vi "CH_LM Config Speedup.vi"(0 "Meter Index":i32, 2 "Speedup Mode (0)":T1, 3 "Status (On)":bool=TRUE, 5 "error in (no error)":errorcluster, 7 "Timeout / ms (3000)":i32=3000, 8 "Action (query)":bool, 9 "Lock Timeout / ms (1000)":i32=1000) -> (11 "Lock timed out":bool, 14 "Meter Index":i32, 17 "Status":bool, 19 "error out":errorcluster)   [LabVIEW 2012, in "CH_LM.lvlib"]
doc: "This command will set/query speedup modes."
uses:
  CH_LM.lvlib
  CH_LM Speedup Type.ctl
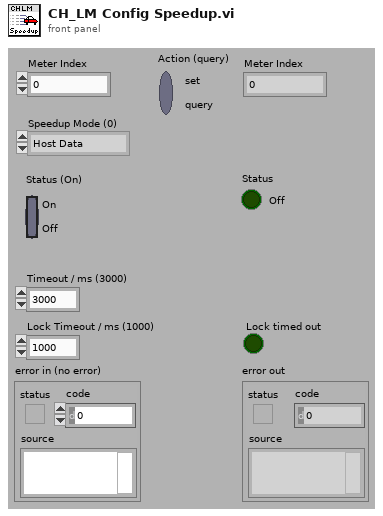
[diagram p1: front panel]
types:
  T1 = typedef "CH_LM.lvlib/CH_LM Speedup Type.ctl" = enum16{"Host Data", "Analog Output", "Numeric Display", "Tune Display"}
  T2 = enum16{"Host Data", "Analog Output", "Numeric Display", "Tune Display"}
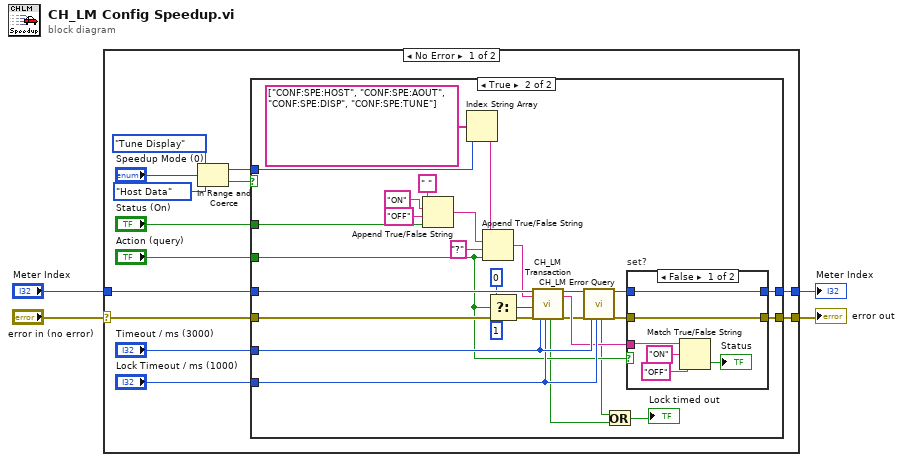
[diagram p0: block diagram]
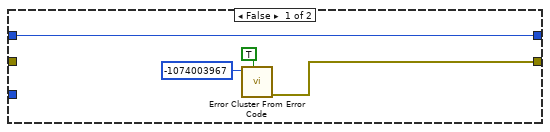
[diagram p2: hidden frame]
diagram:
  n1 = case shown="No Error" "error in (no error)" {
    selector: "error in (no error)" -> [w17 w59]
    tunnel: [w15 w59] -> w4
    tunnel: "Meter Index" -> [w16 w58]
    tunnel: [w14 w58] -> w1
    frame No Error {
      n2 = In Range and Coerce(upper limit=T2."Tune Display", x="Speedup Mode (0)", lower limit=T2."Host Data") -> (coerced(x)=w8:T1, In Range?=w5:bool)
      n3 = case shown="True" w5 {
        tunnel: w17 -> [_ w49]
        tunnel: w16 -> [w21 w48]
        tunnel: [w18 w47] -> w15
        tunnel: [w21 w46] -> w14
        tunnel: "Timeout / ms (3000)" -> [_ w45]
        tunnel: "Lock Timeout / ms (1000)" -> [_ w44]
        tunnel: "Action (query)" -> [_ w43]
        tunnel: "Status (On)" -> [_ w28]
        tunnel: w8 -> [_ w22]
        frame False {
          n4 = call <vilib>:"Error Cluster From Error Code.vi"("show call chain? (False)"=TRUE, "error code (0)"=-1074003967) -> ("error out"=w18:errorcluster)  [unwired: 1 in, 6 out]
        }
        frame True {
          n5 = Append True/False String(1:w28, 2:"OFF" ("false string"), 3:"ON" ("true string"), 4:" ") -> (0:w23:string)
          n6 = Index String Array(1:w22, 2:string[] ["CONF:SPE:HOST", "CONF:SPE:AOUT", "CONF:SPE:DISP", "CONF:SPE:TUNE"]) -> (0:w29:string)  [unwired: 1 out]
          n7 = Append True/False String(1:w43, 2:"?" ("true string"), 3:w23, 4:w29) -> (0:w25:string)
          n8 = Select(t=0, s=w43, f=1 ("NofStrings (-1:all)")) -> (s? t:f=w39:i32)
          n9 = call "CH_LM Transaction.vi"("Meter Index"=w48, "Command String"=w25, "NofStrings (-1:all)"=w39, "error in (no error)"=w49, "Timeout / ms (3000)"=w45, "Lock Timeout / ms (1000)"=w44) -> ("Lock timed out"=w32:bool, "Meter Index"=w37:i32, "Response"=w42:string, "error out"=w35:errorcluster)  [unwired: 10 out]
          n10 = call "CH_LM Error Query.vi"("Meter Index"=w37, "error in (no error)"=w35, "Timeout / ms (3000)"=w45, "Lock Timeout / ms (1000)"=w44) -> ("Lock timed out"=w33:bool, "Meter Index"=w36:i32, "error out"=w34:errorcluster)  [unwired: 13 out]
          n11 = Or(x=w33, y=w32) -> (x .or. y?=→"Lock timed out":bool)
          n12 = case "set?" shown="False" w43 {
            tunnel: w42 -> [w53 _]
            tunnel: w34 -> [w54 w57]
            tunnel: [w54 w57] -> w47
            tunnel: w36 -> [w55 w56]
            tunnel: [w55 w56] -> w46
            frame False {
              n13 = Match True/False String(2:"OFF" ("false string"), 3:"ON" ("true string"), 4:w53) -> (0:→"Status":bool)  [unwired: 1 out]
            }
            frame True {
            }
          }
        }
      }
    }
    frame Error {
    }
  }
  "error out" <- w4
  "Meter Index" <- w1
